vi "그래프 저장_Test.vi"() -> ()   [LabVIEW 2024]
uses:
  <vilib>/Utility/sysdir.llb/System Directory Type.ctl
panel:
  out "웨이브폼 차트 4":dbl[](graph)
  out "웨이브폼 차트 3":dbl[](graph)
  out "웨이브폼 차트 2":dbl[](graph)
  in  "정지":bool
  in  "버튼":bool
  out "웨이브폼 차트":dbl[](graph)
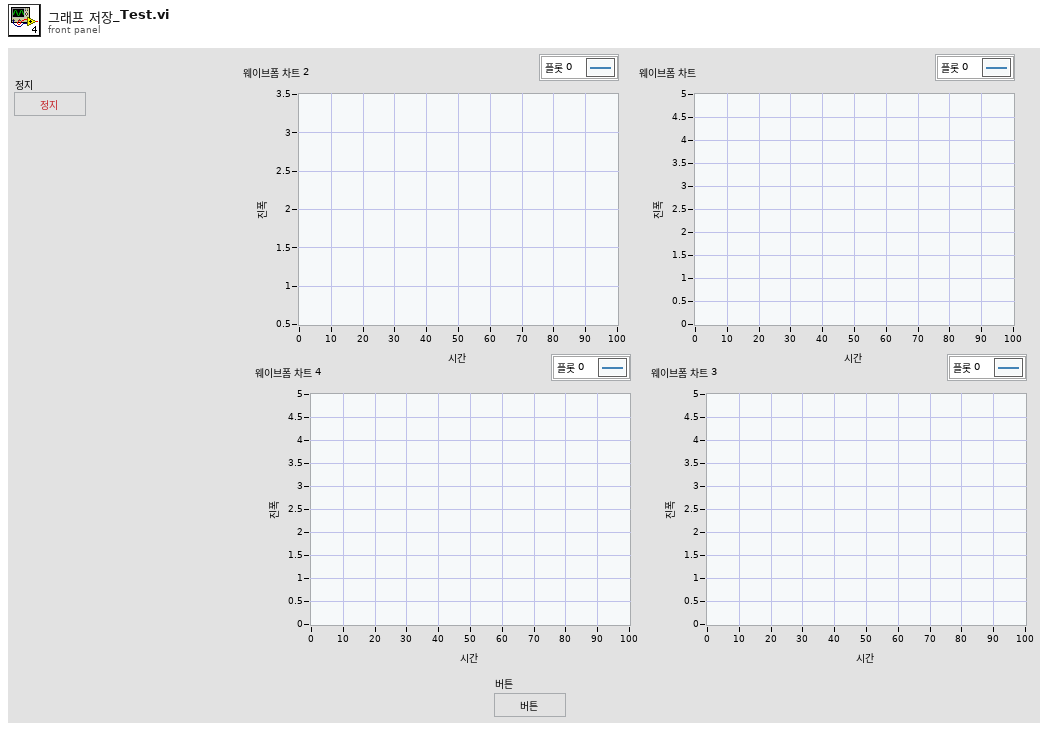
[diagram p1: front panel]
types:
  T1 = typedef "System Directory Type.ctl" = i32
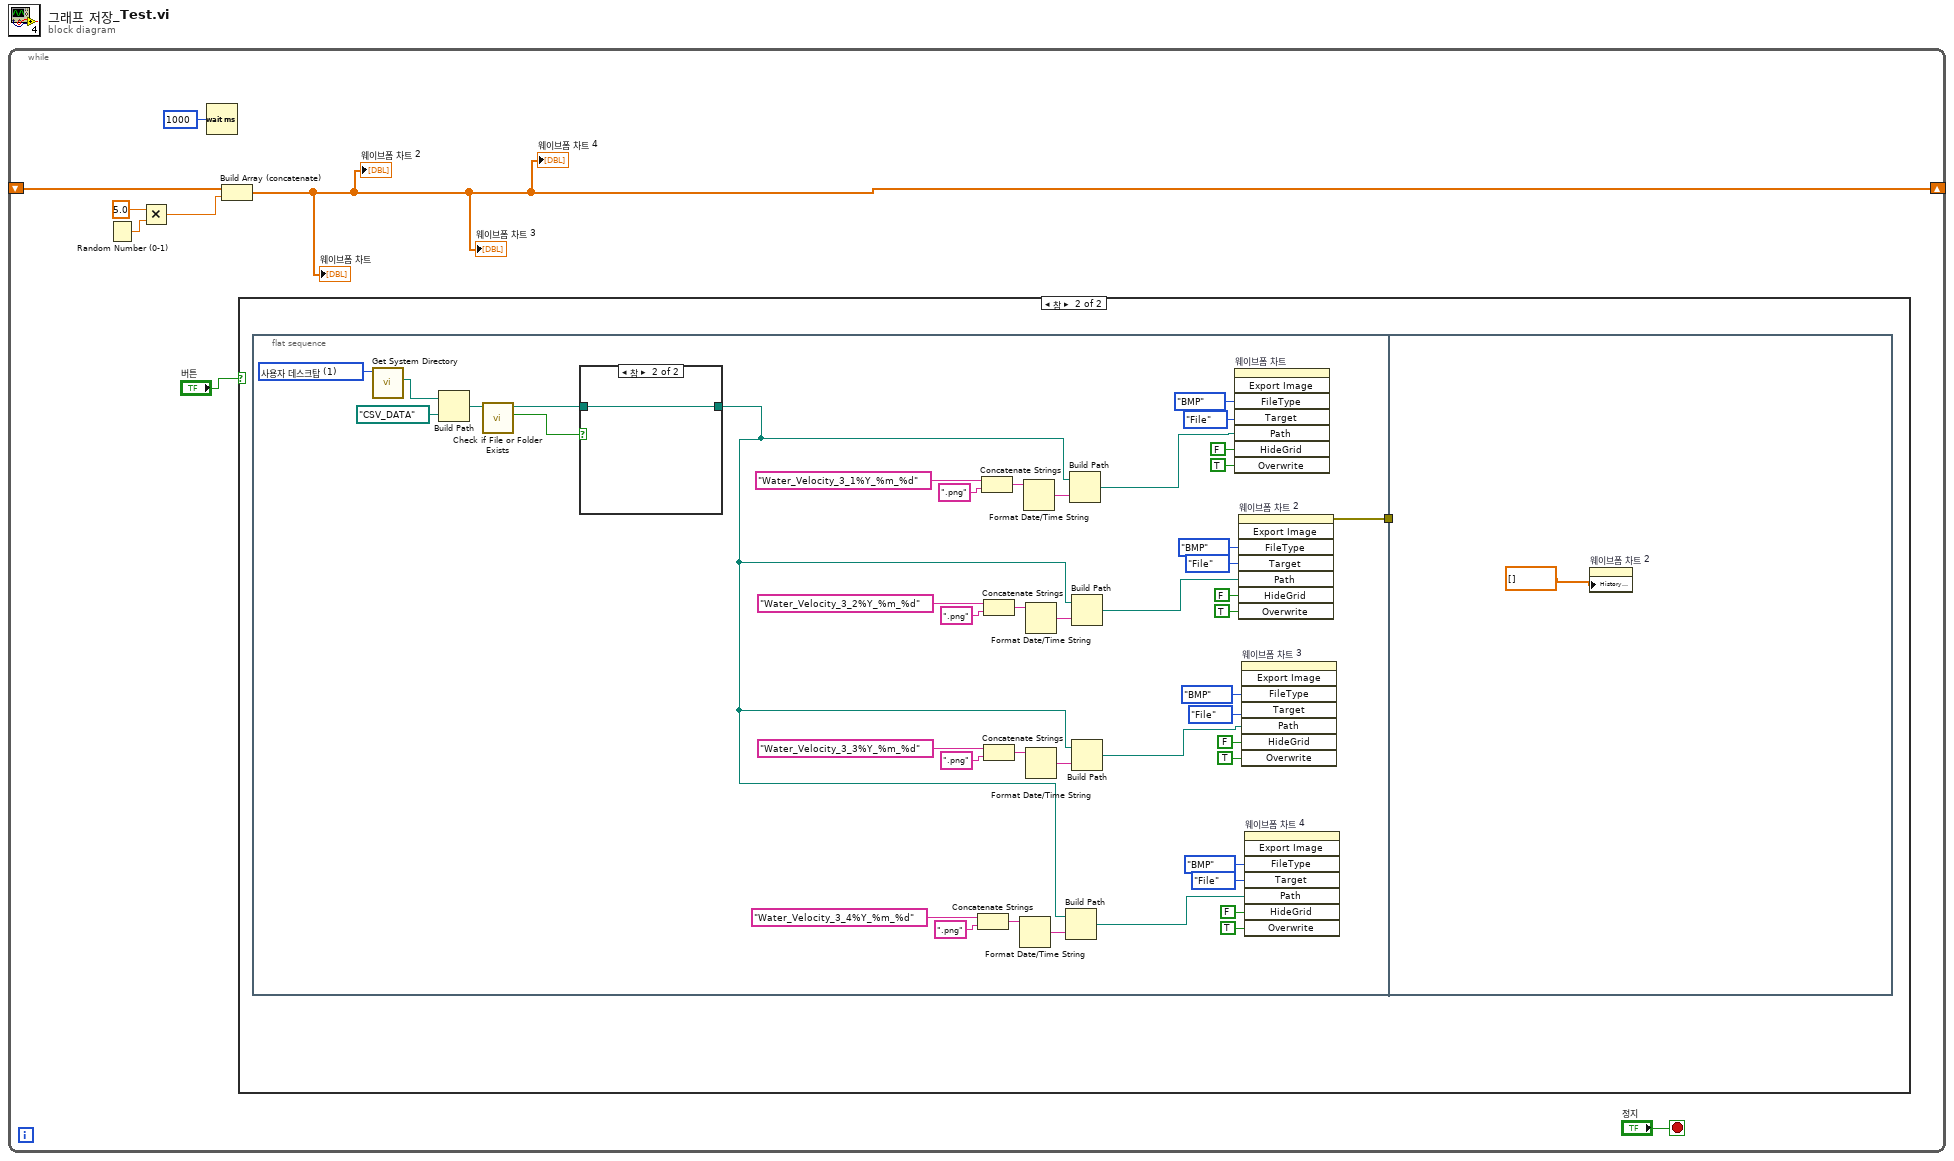
[diagram p0: block diagram]
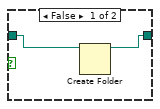
[diagram p3: hidden frame]
diagram:
  n1 = while {
    shift-right: [w1] -> _
    shift-left: _ -> [w6]
    stop <- "정지" stop-if-true
    n2 = Random Number (0-1)() -> (number: 0 to 1=w8:dbl)
    n3 = Multiply(x=5.0, y=w8) -> (x*y=w5:dbl)
    n4 = Wait (ms)(milliseconds to wait=u32 1000 ("대기 시간 (ms)")) -> ()  [unwired: 1 out]
    n5 = Build Array (concatenate)(w6, w5) -> (w1:dbl[])
    "웨이브폼 차트" <- w1
    "웨이브폼 차트 2" <- w1
    "웨이브폼 차트 4" <- w1
    "웨이브폼 차트 3" <- w1
    n6 = case shown="참" "버튼" {
      frame False {
      }
      frame True {
        n7 = flat-sequence {
          tunnel: [w10] -> w9
          tunnel: w9 -> [_]
          frame #0 {
            w51 = T1 1 items=["사용자 홈"=0, "사용자 데스크탑"=1, "사용자 문서"=2, "사용자 어플리케이션 데이터"=3, "사용자 환경"=4, "사용자 임시"=5, "퍼블릭 문서"=6, "퍼블릭 어플리케이션 데이터"=7, "퍼블릭 환경"=8, "퍼블릭 캐시"=13, "시스템 코어 라이브러리"=9, "시스템 설치된 라이브러리"=10, "어플리케이션 파일"=11, "부팅 볼륨 루트"=12] ("system directory type")
            n8 = call <vilib>:"Get System Directory.vi"("system directory type"=w51) -> ("system directory"=w50:path)  [unwired: 10 in]
            n9 = Build Path(base path=w50, name or relative path=path "CSV_DATA" ("이름 또는 상대 경로")) -> (appended path=w48:path)
            n10 = call <vilib>:"Check if File or Folder Exists.vi"("path"=w48) -> ("file or folder exists?"=w47:bool, "dup path"=w46:path)  [unwired: 8 in, 1 out]
            n11 = case shown="참" w47 {
              tunnel: [w54 w56] -> w15
              tunnel: w46 -> [w55 w56]
              frame False {
                n12 = Create Folder(path (use dialog)=w55) -> (created path=w54:path)  [unwired: 2 in, 2 out]
              }
              frame True {
              }
            }
            n13 = Concatenate Strings("Water_Velocity_3_4%Y_%m_%d" ("시간 포맷 문자열 (%c)"), ".png" ("시간 포맷 문자열 (%c)")) -> (w18:string)
            n14 = Concatenate Strings("Water_Velocity_3_1%Y_%m_%d" ("시간 포맷 문자열 (%c)"), ".png" ("시간 포맷 문자열 (%c)")) -> (w29:string)
            n15 = Concatenate Strings("Water_Velocity_3_2%Y_%m_%d" ("시간 포맷 문자열 (%c)"), ".png" ("시간 포맷 문자열 (%c)")) -> (w26:string)
            n16 = Concatenate Strings("Water_Velocity_3_3%Y_%m_%d" ("시간 포맷 문자열 (%c)"), ".png" ("시간 포맷 문자열 (%c)")) -> (w21:string)
            n17 = Format Date/Time String(time format string (%c)=w18) -> (date/time string=w19:string)  [unwired: 2 in]
            n18 = Format Date/Time String(time format string (%c)=w29) -> (date/time string=w28:string)  [unwired: 2 in]
            n19 = Format Date/Time String(time format string (%c)=w26) -> (date/time string=w27:string)  [unwired: 2 in]
            n20 = Format Date/Time String(time format string (%c)=w21) -> (date/time string=w20:string)  [unwired: 2 in]
            n21 = Build Path(base path=w15, name or relative path=w19) -> (appended path=w11:path)
            n22 = Build Path(base path=w15, name or relative path=w28) -> (appended path=w14:path)
            n23 = Build Path(base path=w15, name or relative path=w27) -> (appended path=w13:path)
            n24 = Build Path(base path=w15, name or relative path=w20) -> (appended path=w12:path)
            n25 = invoke on="웨이브폼 차트" class="WFChart (엄격한)" method="Export Image"("FileType"=enum32{"BMP", "EPS", "EMF", "PICT"}."BMP" ("파일 타입"), "Target"=enum32{"File", "Clipboard"}."File" ("타겟"), "Path"=w14, "HideGrid"=FALSE ("눈금 숨기기"), "Overwrite"=TRUE ("항상 덮어쓰기")) -> ()  [unwired: 3 in, 8 out]
            n26 = invoke on="웨이브폼 차트 2" class="WFChart (엄격한)" method="Export Image"("FileType"=enum32{"BMP", "EPS", "EMF", "PICT"}."BMP" ("파일 타입"), "Target"=enum32{"File", "Clipboard"}."File" ("타겟"), "Path"=w13, "HideGrid"=FALSE ("눈금 숨기기"), "Overwrite"=TRUE ("항상 덮어쓰기")) -> (error out=w10:errorcluster)  [unwired: 3 in, 7 out]
            n27 = invoke on="웨이브폼 차트 3" class="WFChart (엄격한)" method="Export Image"("FileType"=enum32{"BMP", "EPS", "EMF", "PICT"}."BMP" ("파일 타입"), "Target"=enum32{"File", "Clipboard"}."File" ("타겟"), "Path"=w12, "HideGrid"=FALSE ("눈금 숨기기"), "Overwrite"=TRUE ("항상 덮어쓰기")) -> ()  [unwired: 3 in, 8 out]
            n28 = invoke on="웨이브폼 차트 4" class="WFChart (엄격한)" method="Export Image"("FileType"=enum32{"BMP", "EPS", "EMF", "PICT"}."BMP" ("파일 타입"), "Target"=enum32{"File", "Clipboard"}."File" ("타겟"), "Path"=w11, "HideGrid"=FALSE ("눈금 숨기기"), "Overwrite"=TRUE ("항상 덮어쓰기")) -> ()  [unwired: 3 in, 8 out]
          }
          frame #1 {
            n29 = property on="웨이브폼 차트 2" class="WFChart (엄격한)"("History Data"=dbl[] [] ("값(신호)")) -> ()  [unwired: 2 in, 2 out]
          }
        }
      }
    }
  }
